vi "Write Array.vi"(10 "Array":T1[](array[typedef]), 11 "CCD in":refnum<class "CCD.lvclass">) -> (3 "CCD out":refnum<class "CCD.lvclass">)   [LabVIEW 2016, in "Hardware.lvlib" / "CCD.lvlib" / "CCD.lvclass"]
uses:
  <userlib>/Common Components/Hardware/CCD/CCD/CCD.lvclass
  <vilib>/userdefined/High Color/IMAQdx.ctl
  <userlib>/Common Components/Hardware/CCD/CCD/CCD.lvclass/CCD.ctl
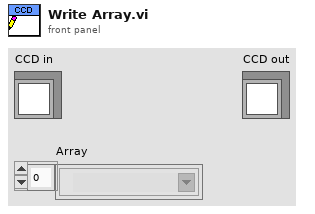
[diagram p1: front panel]
types:
  T1 = typedef "IMAQdx.ctl" = refnum<k21>
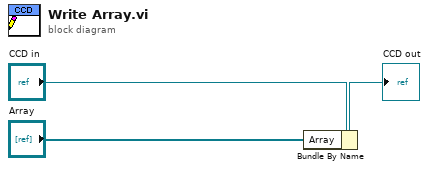
[diagram p0: block diagram]
diagram:
  n1 = Bundle By Name(cluster="CCD in", "Array"="Array") -> (→"CCD out":refnum<class "CCD.lvclass">)
